vi "Pressure Read.vi"() -> ()   [LabVIEW 2018]
uses:
  <vilib>/DAQmx/read.llb/DAQmx Read (Analog Wfm 1Chan 1Samp).vi
  <vilib>/DAQmx/create/channels.llb/DAQmx Create Channel (AI-Current-Basic).vi
  <vilib>/DAQmx/miscellaneous.llb/DAQmx Fill In Error Info.vi
panel:
  out "data":waveform(dbl)
  out "Waveform Chart":waveform(dbl)(graph)
  in  "physical channels":tag="cDAQ2Mod8/ai15"
  in  "name to assign":string="Pressure 1"
  in  "stop":bool
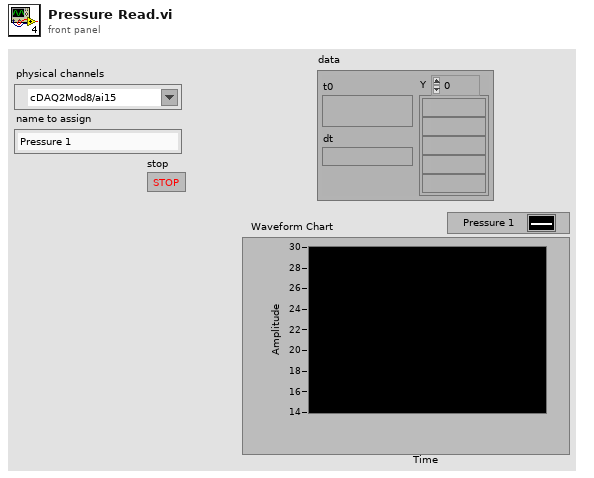
[diagram p1: front panel]
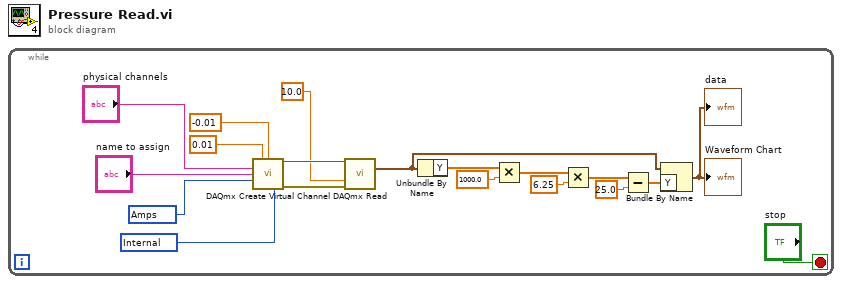
[diagram p0: block diagram]
diagram:
  n1 = while {
    stop <- "stop" stop-if-true
    w10 = 10200 items=["default"=-1, "Internal"=10200, "External"=10167] ("shunt resistor location")
    w11 = 10342 items=["Amps"=10342, "From Custom Scale"=10065] ("units")
    n2 = call-poly <vilib>:"DAQmx Create Virtual Channel.vi"("maximum value"=0.01, "minimum value"=-0.01, "physical channels"="physical channels", "name to assign"="name to assign", "units"=w11, "shunt resistor location"=w10) -> ("task out"=w19:refnum<k21>, "error out"=w18:errorcluster)  [unwired: 8 in]
    n3 = call-poly <vilib>:"DAQmx Read.vi"("task/channels in"=w19, "timeout"=10.0, "error in"=w18) -> ("data"=w4:waveform(dbl))  [unwired: 10 in, 2 out]
    n4 = Unbundle By Name(w4) -> ("Y"=w2:dbl[])
    n5 = Multiply(x=w2, y=1000.0) -> (x*y=w3:dbl[])
    n6 = Multiply(x=w3, y=6.25) -> (x*y=w7:dbl[])
    n7 = Subtract(x=w7, y=25.0) -> (x-y=w6:dbl[])
    n8 = Bundle By Name(cluster=w4, "Y"=w6) -> (→"Waveform Chart" →"data":waveform(dbl))
  }
